vi "Get Type.vi"(0 "image in":refnum<class "MSC Image.lvclass">, 5 "error in (no error)":errorcluster) -> (14 "image out":refnum<class "MSC Image.lvclass">, 15 "Image Type":T1 items=["Grayscale U8"=0, "Grayscale U16"=2, "Grayscale Single"=5, "Grayscale Double"=6, "RGB U8"=16], 19 "error out":errorcluster)   [LabVIEW 2014, in "MSC Image.lvclass"]
doc: "Returns the image type."
uses:
  MSC Image.lvclass
  controls/Image Type.ctl
  MSC Image.lvclass/MSC Image.ctl
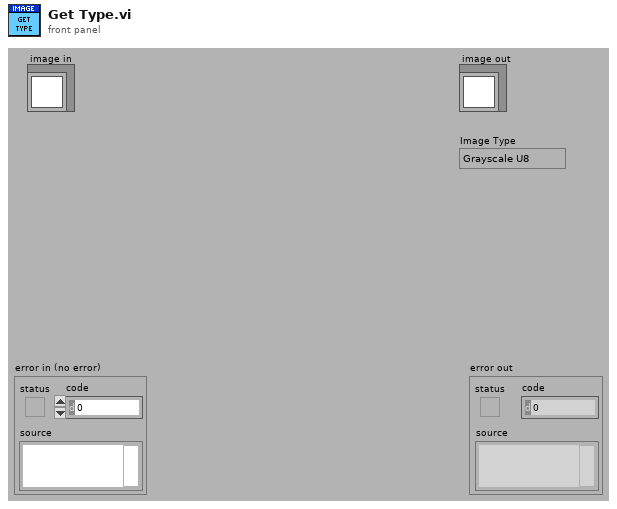
[diagram p1: front panel]
types:
  T1 = typedef "MSC Image.lvclass/Image Type.ctl" = i32
  T2 = typedef "Image.ctl" = cluster{"Pointer":u64, "Size":T3, "Image Type":T4, "Time Stamp":timestamp, "Variant":variant}
  T3 = typedef "Size.ctl" = cluster{"Cols":i32, "Rows":i32}
  T4 = typedef "Image Type.ctl" = i32
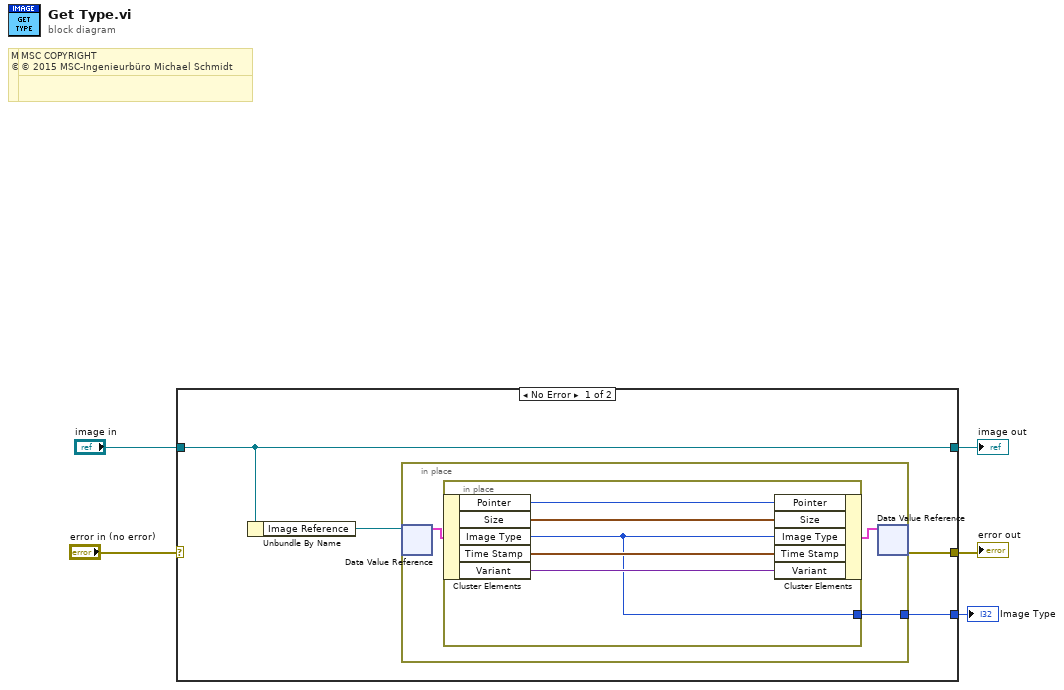
[diagram p0: block diagram]
diagram:
  # "MSC COPYRIGHT\n© 2016 MSC-Ingenieurbüro Michael Schmidt"
  # "MSC COPYRIGHT\n© 2016 MSC-Ingenieurbüro Michael Schmidt"
  # "MSC COPYRIGHT\n© 2015 MSC-Ingenieurbüro Michael Schmidt"
  # "MSC COPYRIGHT\n© 2015 MSC-Ingenieurbüro Michael Schmidt"
  n1 = case shown="No Error" "error in (no error)" {
    selector: "error in (no error)" -> [_ w19]
    tunnel: [w7 w19] -> w4
    tunnel: [w9 w18] -> w2
    tunnel: "image in" -> [w9 w18]
    tunnel: [w6 _] -> w1
    frame No Error {
      n2 = Unbundle By Name(w9) -> ("Image Reference"=w8:refnum<data-value>)
      n3 = in-place {
        in-place-border: [w10] -> w6
        n4 = in-place-dvr #1(w8) -> (w11:T2)  [unwired: 1 out]
        n5 = in-place {
          in-place-border: [w13] -> w10
          n6 = in-place-cluster #2(w11) -> ("Pointer"=w17:u64, "Size"=w14:T3, "Image Type"=w13:T4, "Time Stamp"=w15:timestamp, "Variant"=w16:variant)
          n7 = in-place-cluster #2("Pointer"=w17, "Size"=w14, "Image Type"=w13, "Time Stamp"=w15, "Variant"=w16) -> (w12:T2)
        }
        n8 = in-place-dvr #1(w12) -> (w7:errorcluster)  [unwired: 1 out]
      }
    }
    frame Error {
    }
  }
  "error out" <- w4
  "image out" <- w2
  "Image Type" <- w1
